vi "GainFunction.vi"(8 "Velocity":dbl, 11 "Interpolate":bool) -> (3 "PID gains":cluster{"P":dbl, "I":dbl, "D":dbl})   [LabVIEW 2016]
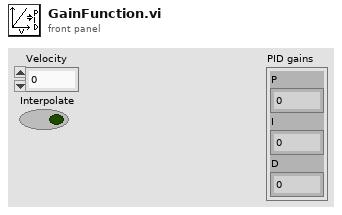
[diagram p1: front panel]
types:
  T1 = cluster{"Proportional gain (Kc)":dbl, "Integral time (Ti, min)":dbl, "Derivative time (Td, min)":dbl}
  T2 = cluster{"upper limit":dbl, "upper limit":dbl, "upper limit":dbl}
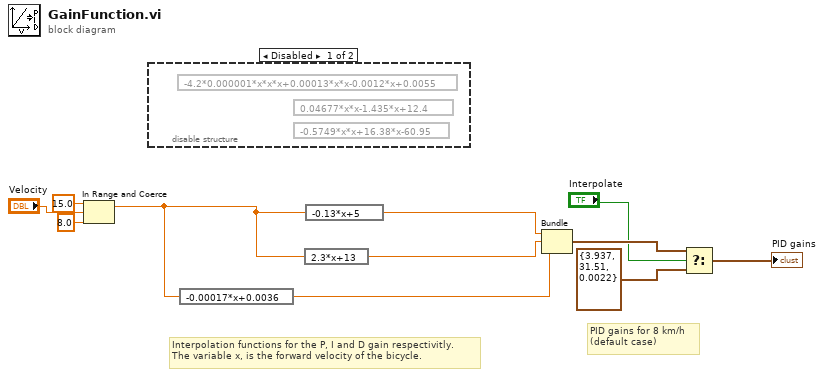
[diagram p0: block diagram]
diagram:
  # "PID gains for 8 km/h\n(default case)"
  # "Interpolation functions for the P, I and D gain respectivitly.\nThe variable x, is the forward velocity of the bicycle."
  n1 = In Range and Coerce(upper limit=15.0, x="Velocity", lower limit=8.0) -> (coerced(x)=w4:dbl)  [unwired: 1 out]
  n2 = disable-structure shown="Disabled" {
    frame Disabled {
      n3 = expression code="-4.2*0.000001*x*x*x+0.00013*x*x-0.0012*x+0.0055"() -> ()  [unwired: 1 in, 1 out]
      n4 = expression code="0.04677*x*x-1.435*x+12.4"() -> ()  [unwired: 1 in, 1 out]
      n5 = expression code="-0.5749*x*x+16.38*x-60.95"() -> ()  [unwired: 1 in, 1 out]
    }
    frame Enabled {
    }
  }
  n6 = expression code="-0.00017*x+0.0036"(w4) -> (w9:dbl)
  n7 = expression code="2.3*x+13"(w4) -> (w10:dbl)
  n8 = expression code="-0.13*x+5"(w4) -> (w11:dbl)
  n9 = Bundle("upper limit"=w11, "upper limit"=w10, "upper limit"=w9) -> (w8:T2)  [unwired: 1 in]
  n10 = Select(t=w8, s="Interpolate", f=T1 {"Proportional gain (Kc)"=3.937, "Integral time (Ti, min)"=31.51, "Derivative time (Td, min)"=0.0022} ("8km/h PID gains")) -> (s? t:f=→"PID gains":T1)
